vi "Bang_Bang_LOX_1.vi"() -> ()   [LabVIEW 2019]
panel:
  in  "test":dbl
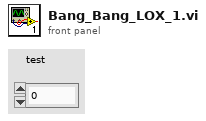
[diagram p1: front panel]
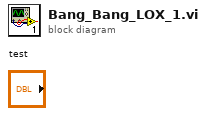
[diagram p0: block diagram]
diagram:
